vi "Encoder to Normalized Velocity.vi"(11 "ticks/100ms":dbl) -> (3 "ft/s":dbl)   [LabVIEW 2018]
doc: "Converting ticks/100ms to ft/s given drive base information"
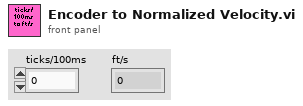
[diagram p1: front panel]
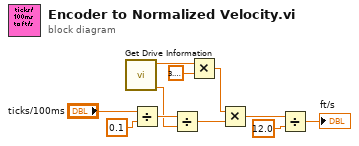
[diagram p0: block diagram]
diagram:
  n1 = call "Get Drive Information.vi"() -> ("Ticks/Revolution"=w1:dbl, "Wheel Diameter"=w2:dbl)  [unwired: 10 in]
  n2 = Divide(x="ticks/100ms", y=0.1) -> (x/y=w9:dbl)
  n3 = Divide(x=w9, y=w1) -> (x/y=w8:dbl)
  n4 = Multiply(x=w2, y=3.141592653589793) -> (x*y=w6:dbl)
  n5 = Multiply(x=w6, y=w8) -> (x*y=w5:dbl)
  n6 = Divide(x=w5, y=12.0) -> (x/y=→"ft/s":dbl)
